vi "get_buf.vi"(4 "error in":errorcluster, 5 "Sync cluster":T2, 6 "acquisition status":i32, 7 "Scope Cluster":T1) -> (0 "error out":errorcluster, 1 "wfm":waveform(i16)[](array[waveform]), 2 "acquisition status out":i32 caption="acquisition status")   [LabVIEW 2010]
uses:
  lib/Global 2.vi
  <instrlib>/niSync/niSync.llb/niSync Read Trigger Time Stamp (Multiple).vi
  <instrlib>/niScope/Acquire/niScope Multi Read WDT.vi
  <instrlib>/niScope/Acquire/Fetch/niScope Multi Fetch WDT.vi
panel:
  out "fetch":bool
  out "Available Stamps":i32
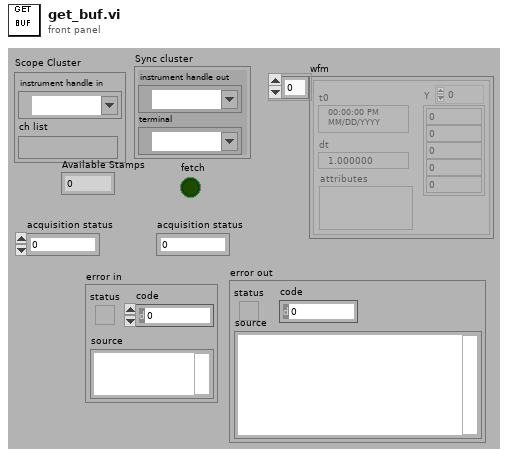
[diagram p1: front panel]
types:
  T1 = cluster{"instrument handle in":refnum<k15>, "ch list":string}
  T2 = cluster{"instrument handle out":refnum<k15>, "terminal":tag}
  T3 = cluster{"name":enum16{"sync", "phase_a", "phase_b", "phase_c", "ground"}, "num":i32}[]
  T4 = enum16{"sync", "phase_a", "phase_b", "phase_c", "ground"}
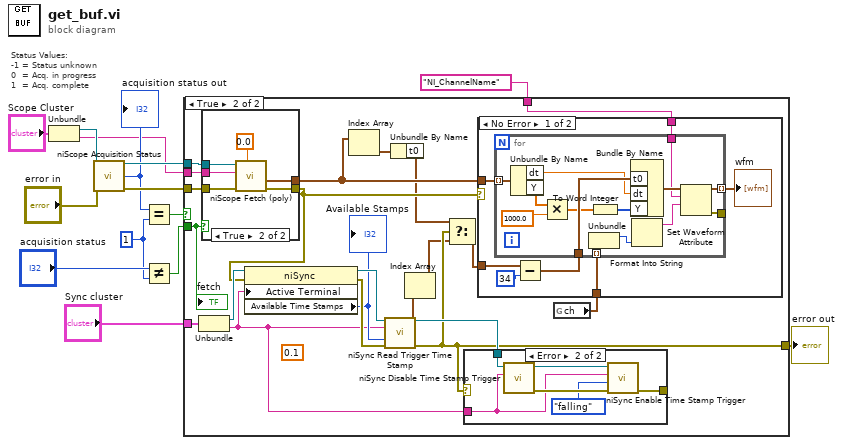
[diagram p0: block diagram]
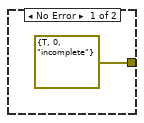
[diagram p3: hidden frame]
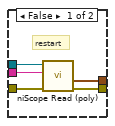
[diagram p6: hidden frame]
diagram:
  w7 = 1 ("y")
  # "Status Values:\n-1 = Status unknown\n0  = Acq. in progress\n1  = Acq. complete"
  n1 = Unbundle("Scope Cluster") -> ("instrument handle in"=w4:refnum<k15>, "ch list"=w3:string)
  n2 = call <instrlib>:"niScope Acquisition Status.vi"("instrument handle"=w4, "error in"="error in") -> ("instrument handle out"=w14:refnum<k15>, "acquisition status"=w11:i32, "error out"=w13:errorcluster)  [unwired: 11 in]
  "acquisition status out" <- w11
  n3 = Equal?(x=w11, y=w7) -> (x = y?=w9:bool)
  n4 = Not Equal?(x="acquisition status", y=w7) -> (x != y?=w8:bool)
  n5 = case shown="True" w9 {
    tunnel: w14 -> [_ w39]
    tunnel: w13 -> [w15 w38]
    tunnel: [w16 w22] -> w1
    tunnel: w8 -> [_ w28]
    tunnel: "Sync cluster" -> [_ w37]
    tunnel: w3 -> [_ w36]
    tunnel: "NI_ChannelName" ("name") -> [_ w35]
    frame False {
      n6 = case shown="Error" w15 {
        selector: w15 -> [_ w18]
        tunnel: [errorcluster {"status"=TRUE, "code"=0, "source"="incomplete"} ("error out") w18] -> w16
        frame No Error {
        }
        frame Error {
        }
      }
    }
    frame True {
      (unwired) 0.1 ("timeout")
      n7 = Unbundle(w37) -> ("instrument handle out"=w33:refnum<k15>, "terminal"=w25:tag)
      n8 = case shown="True" w28 {
        tunnel: w39 -> [w70 w77]
        tunnel: w38 -> [w72 w76]
        tunnel: [w69 w75] -> w27
        tunnel: [w68 w74] -> w24
        tunnel: w36 -> [w71 w73]
        frame False {
          # "restart"
          n9 = call-poly <instrlib>:"niScope Read (poly).vi"("error in"=w72, "channels"=w71, "instrument handle"=w70) -> ("error out"=w69:errorcluster, "wfm"=w68:waveform(dbl)[])  [unwired: 5 in, 2 out]
        }
        frame True {
          n10 = call-poly <instrlib>:"niScope Fetch (poly).vi"("timeout"=0.0, "error in"=w76, "channels"=w73, "instrument handle"=w77) -> ("error out"=w75:errorcluster, "wfm"=w74:waveform(dbl)[])  [unwired: 4 in, 2 out]
        }
      }
      n11 = property class="niSync"(reference=w33, error in=w27, "Active Terminal"=w25) -> (reference out=w32:refnum<k15>, error out=w31:errorcluster, "Available Time Stamps"=w29:i32)
      "Available Stamps" <- w29
      n12 = Index Array(array=w24) -> (element=w23:waveform(dbl))  [unwired: 1 in]
      n13 = call-poly <instrlib>:"niSync Read Trigger Time Stamp.vi"("instrument handle"=w32, "terminal"=w25, "number of timestamps"=w29, "error in (no error)"=w31) -> ("instrument handle out"=w26:refnum<k15>, "time stamp out"=w30:timestamp[], "error out"=w22:errorcluster)  [unwired: 8 in, 1 out]
      n14 = Unbundle By Name(w23) -> ("t0"=w21:timestamp)
      n15 = Index Array(array=w30) -> (element=w20:timestamp)  [unwired: 1 in]
      n16 = Select(t=w21, s=w22, f=w20) -> (s? t:f=w19:timestamp)
      n17 = case shown="Error" w22 {
        selector: w22 -> [w40 _]
        tunnel: w26 -> [_ w44]
        tunnel: w25 -> [_ w43]
        tunnel: [w40 w41] -> _
        frame No Error {
        }
        frame Error {
          n18 = call <instrlib>:"niSync Disable Time Stamp Trigger.vi"("terminal"=w43, "instrument handle"=w44) -> ("error out"=w46:errorcluster, "instrument handle out"=w45:refnum<k15>)  [unwired: 7 in]
          n19 = call <instrlib>:"niSync Enable Time Stamp Trigger.vi"("error in (no error)"=w46, "active edge"=enum32{"rising", "falling", "any"}."falling", "terminal"=w43, "instrument handle"=w45) -> ("error out"=w41:errorcluster)  [unwired: 5 in, 1 out]
        }
      }
      n20 = global read "Global 2.vi" "ch"() -> (w34:T3)
      n21 = case shown="No Error" w27 {
        tunnel: w24 -> [w53 _]
        tunnel: w19 -> [w50 _]
        tunnel: w35 -> [w49 _]
        tunnel: w34 -> [w48 _]
        frame No Error {
          n22 = Subtract(x=w50, y=34) -> (x-y=w51:timestamp)
          n23 = for {
            tunnel: w53 -> [w66] mode=indexing
            tunnel: w51 -> [w67]
            tunnel: [w64] -> w47 mode=indexing
            tunnel: [w63] -> _
            tunnel: w49 -> [w62]
            tunnel: w48 -> [w60] mode=indexing
            n24 = Unbundle By Name(w66) -> ("dt"=w58:dbl, "Y"=w57:dbl[])
            n25 = Multiply(x=w57, y=1000.0) -> (x*y=w56:dbl[])
            n26 = Unbundle(w60) -> ("name"=w59:T4)  [unwired: 1 out]
            n27 = To Word Integer(number=w56) -> (16bit integer=w55:i16[])
            n28 = Bundle By Name("t0"=w67, "dt"=w58, "Y"=w55) -> (w65:waveform(i16))  [unwired: 1 in]
            n29 = Format Into String(w59) -> (resulting string=w61:string)  [unwired: 3 in, 1 out]
            n30 = Set Waveform Attribute(5:w61, 6:w62, 7:w65) -> (0:w63:errorcluster, 3:w64:waveform(i16))  [unwired: 1 in, 1 out]
          }
          "wfm" <- w47
        }
        frame Error {
        }
      }
      "fetch" <- w28
    }
  }
  "error out" <- w1
